vi "GetRunStatus.vi"(0 "Axis In":T3, 11 "error in (no error)":errorcluster) -> (4 "Axis Out":T3, 6 "run status":T1 {"Run Status Description" items=["Fault detected"=1, "Disabled and not faulted"=255, "Enabled"=0]}, 15 "error out":errorcluster)   [LabVIEW 2009]
uses:
  typedefs/AxisSelect_Enum.ctl
  typedefs/Ultra3000/Fault_Cluster.ctl
  typedefs/Ultra3000/RunStatus_Ring.ctl
  typedefs/Ultra3000/Func.ctl
  typedefs/Ultra3000/Cmds.ctl
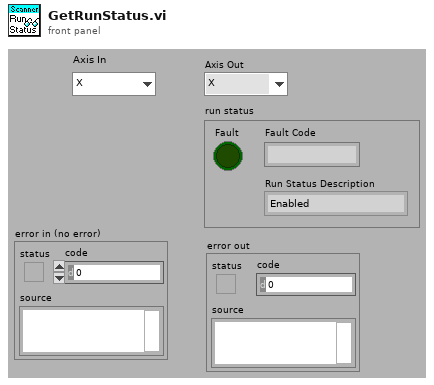
[diagram p1: front panel]
types:
  T1 = typedef "Fault_Cluster.ctl" = cluster{"Fault":bool, "Fault Code":string, "Run Status Description":T2}
  T2 = typedef "RunStatus_Ring.ctl" = u16
  T3 = typedef "AxisSelect_Enum.ctl" = enum16{"X", "Y", "Z", "Axis Space"}
  T4 = typedef "Cmds.ctl" = u16
  T5 = typedef "Func.ctl" = u16
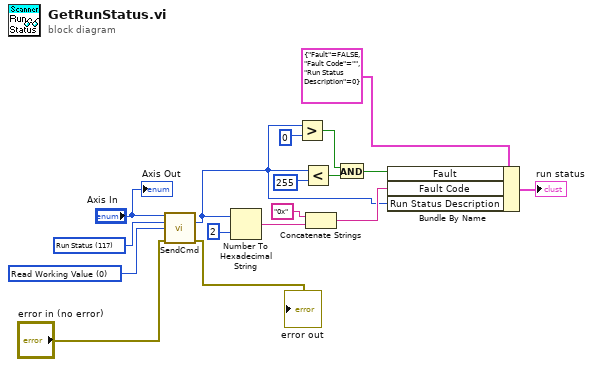
[diagram p0: block diagram]
diagram:
  w5 = T4 117 items=["Run Status"=117, "Fault Status"=116, "Position Error"=129, "Auto-Start Homing"=196, "Start Homing"=205, "Homing Type"=197, "Motor Position"=126, "Velocity Motor"=133, "Power-Up Status"=1, "Drive Name"=6, "Position Window Size"=22, "Position Window Time"=23, "Zero Speed Limit"=34, "Speed Window Size"=35, "Up to Speed Limit"=37, "Forward Current Limit"=47, "Reverse Current Limit"=48, "Override Mode"=67, "Operation Mode"=90, "Host Control Mode"=97, "Reset Drive"=106, "Drive Enable"=107, "Setpoint Current"=108, "Setpoint Velocity"=109, "Setpoint Acceleration"=110, "Reset Faults"=111, "Position Comparator"=349, "Postition Comparator Polarity"=350, "Position Rollover Enable"=404, "Baud Rate"=80, "Frame Format"=81, "Drive Address"=82, "Broadcast Address"=83, "Auto-start Indexing"=88, "Start Index"=112, "Host Index"=184, "Index Type"=174, "Index Dist/Pos"=175, "Index Reg Dist"=176, "Index Velocity"=177, "Index Acceleration"=178, "Index Deceleration"=179, "Index Dwell"=180, "Index Count"=181, "Index Termination"=182, "Index Pointer"=183, "Index Abort Deceleration"=185, "Positive Soft Pos Limit"=216, "Define Home"=113, "Negative Soft Pos Limit"=217] ("Command")
  w17 = T5 0 items=["Read Working Value", "Write Working Value", "Read Non-Volatile Value", "Write Non-Volatile and Woring Value", "Copy Non-Volatile Value to Working Value", "Copy Working Value to Non-Volatile Value", "Read Default Value", "Copy Default Value to Non-Volatile and Working Values", "Read Min Value", "Read Max Value", "Read Array Index Min", "Read Array Index Max"] ("Function")
  n1 = call "SendCmd.vi"("Axis In"="Axis In", "Command"=w5, "Function"=w17, "error in (no error)"="error in (no error)") -> ("Data"=w3:i32, "error out"=→"error out":errorcluster)  [unwired: 8 in, 2 out]
  n2 = Number To Hexadecimal String(1:i16 2 ("width (-)"), 2:w3) -> (0:w11:string)
  n3 = Greater?(x=w3, y=0) -> (0:w14:bool)
  n4 = Less?(x=w3, y=255) -> (x < y?=w13:bool)
  n5 = Concatenate Strings("0x" ("string"), w11) -> (w6:string)
  n6 = And(x=w14, y=w13) -> (x .and. y?=w7:bool)
  n7 = Bundle By Name(cluster=T1 {"Fault"=FALSE, "Fault Code"="", "Run Status Description"=0} ("fault 2"), "Fault"=w7, "Fault Code"=w6, "Run Status Description"=w3) -> (→"run status":T1)
  "Axis Out" <- "Axis In"
